vi "Run.vi"(8 "error in (no error)":errorcluster caption="entrée d'erreur (pas d'erreur)", 11 "Gaussian_Quantiles.lvclass":refnum<class "Gaussian_Quantiles.lvclass">) -> (0 "error out":errorcluster caption="sortie d'erreur", 2 "Data":T1, 3 "Gaussian_Quantiles.lvclass":refnum<class "Gaussian_Quantiles.lvclass">)   [LabVIEW 2020, in "Gaussian_Quantiles.lvclass"]
doc: "Returns :\n\nX : array of shape [n_samples, n_features]\n The generated samples.\n\ny : array of shape [n_samples]\n The integer labels for quantile membership of each sample."
uses:
  Gaussian_Quantiles.lvclass
  Gaussian_Quantiles.lvclass/Gaussian_Quantiles.ctl
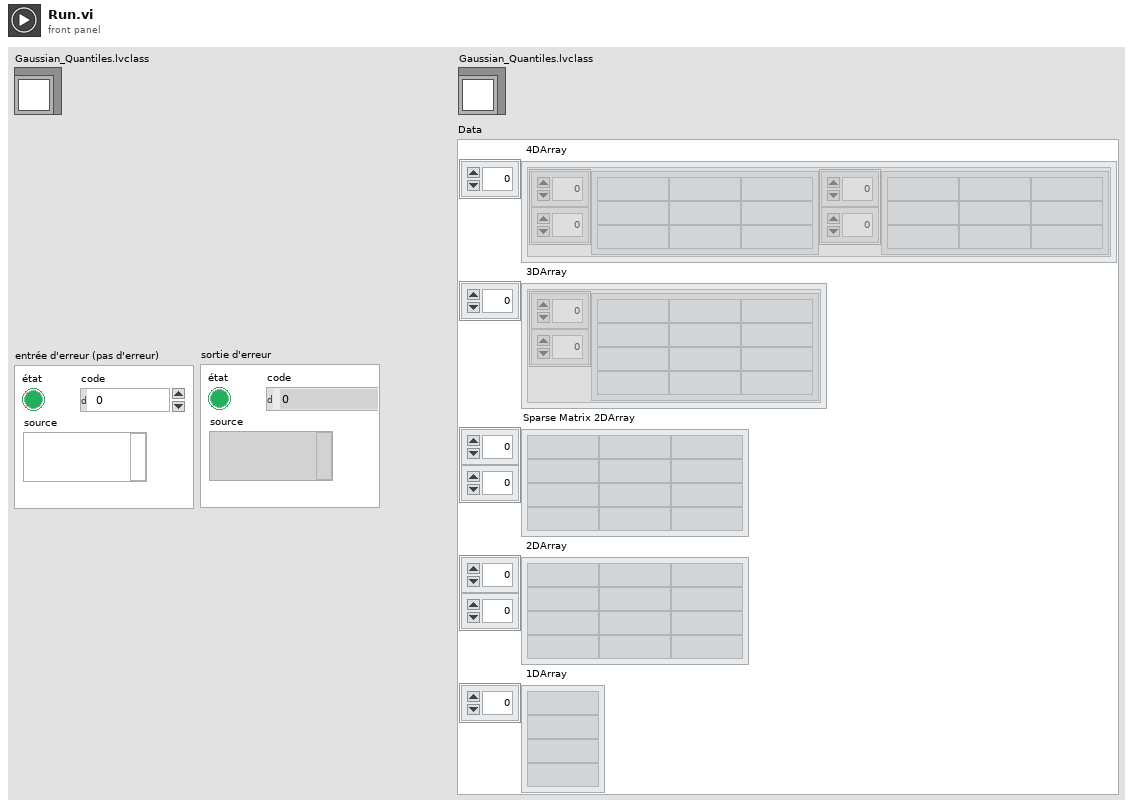
[diagram p1: front panel]
types:
  T1 = cluster{" 4DArray":cluster{"1":string[][], "2":string[][]}[], " 3DArray":cluster{"Tableau":string[][]}[], "Sparse Matrix 2DArray":string[][], " 2DArray":string[][], " 1DArray":string[]}
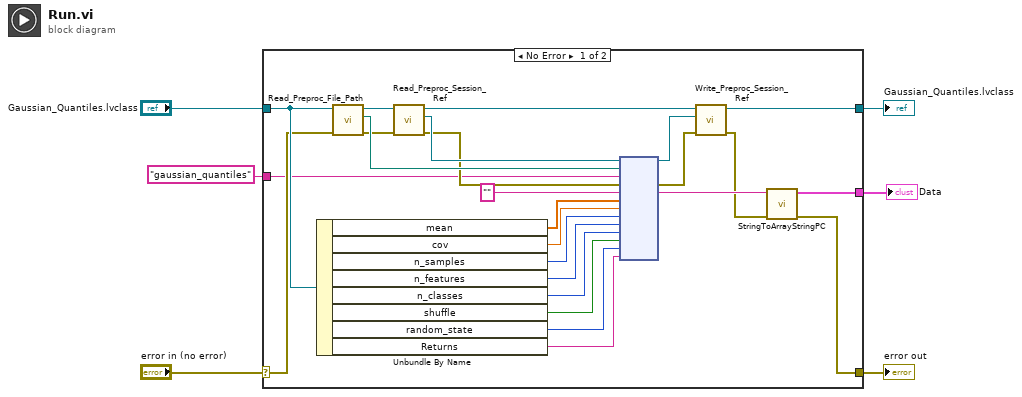
[diagram p0: block diagram]
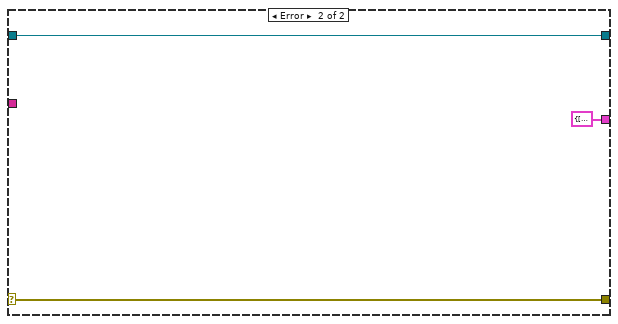
[diagram p2: hidden frame]
diagram:
  n1 = case shown="No Error" "error in (no error)" {
    selector: "error in (no error)" -> [w18 w34]
    tunnel: [w8 w34] -> w5
    tunnel: [w11 w33] -> w3
    tunnel: "Gaussian_Quantiles.lvclass" -> [w19 w33]
    tunnel: "gaussian_quantiles" -> [w17 _]
    tunnel: [w7 T1 {" 4DArray"=[], " 3DArray"=[], "Sparse Matrix 2DArray"=[], " 2DArray"=[], " 1DArray"=[]} ("Data")] -> w1
    frame No Error {
      n2 = Unbundle By Name(w19) -> ("mean"=w22:dbl[], "cov"=w21:dbl, "n_samples"=w20:u32, "n_features"=w16:u32, "n_classes"=w15:u32, "shuffle"=w14:bool, "random_state"=w13:i32, "Returns"=w12:string)
      n3 = call-dynamic "Read_Preproc_File_Path.vi"("error in (no error)"=w18, "Python in"=w19) -> ("error out"=w26:errorcluster, "File_Path"=w29:path, "Python out"=w31:refnum<class "Gaussian_Quantiles.lvclass">)  [unwired: 7 in]
      n4 = call-dynamic "Read_Preproc_Session_Ref.vi"("error in (no error)"=w26, "Python in"=w31) -> ("error out"=w27:errorcluster, "Session_ref"=w28:refnum<k35>, "Python out"=w30:refnum<class "Gaussian_Quantiles.lvclass">)  [unwired: 7 in]
      n5 = node(w28, w29, w17, w27, "", w22, w21, w20, w16, w15, w14, w13, w12) -> (w23:refnum<k35>, w25:errorcluster, w10:string)  [unwired: 8 in, 2 out]
      n6 = call-dynamic "Write_Preproc_Session_Ref.vi"("error in (no error)"=w25, "Session_ref"=w23, "Python in"=w30) -> ("error out"=w9:errorcluster, "Python out"=w11:refnum<class "Gaussian_Quantiles.lvclass">)  [unwired: 7 in]
      n7 = call "StringToArrayStringPC.vi"("sortie d'erreur"=w9, "Return value"=w10) -> ("sortie d'erreur"=w8:errorcluster, "Data"=w7:T1)  [unwired: 8 in]
    }
    frame Error {
    }
  }
  "error out" <- w5
  "Gaussian_Quantiles.lvclass" <- w3
  "Data" <- w1
